vi "AudioStreamer.Get Error Message.vi"() -> (0 "message":string)   [LabVIEW 2020]
uses:
  Typedefs/AudioStreamer.Globals.vi
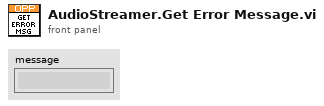
[diagram p1: front panel]
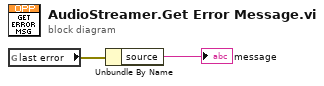
[diagram p0: block diagram]
diagram:
  n1 = global read "AudioStreamer.Globals.vi" "last error"() -> (w2:errorcluster)
  n2 = Unbundle By Name(w2) -> ("source"=→"message":string)
